vi "Calc_frequency.vi"(0 "ExitationTime In":dbl, 1 "X-length":dbl, 5 "CamTolerance":dbl=1.1, 9 "frequency in":dbl=5000.0, 11 "error in":errorcluster, 12 "X-Delta":dbl) -> (2 "Wavepoints":dbl, 3 "N":dbl=8192.0, 4 "TriggerLineCamWavepoints":dbl[](array[numeric]), 6 "divisor out":i32, 8 "Array":u8[](array[numeric]), 15 "error out":errorcluster)   [LabVIEW 2011]
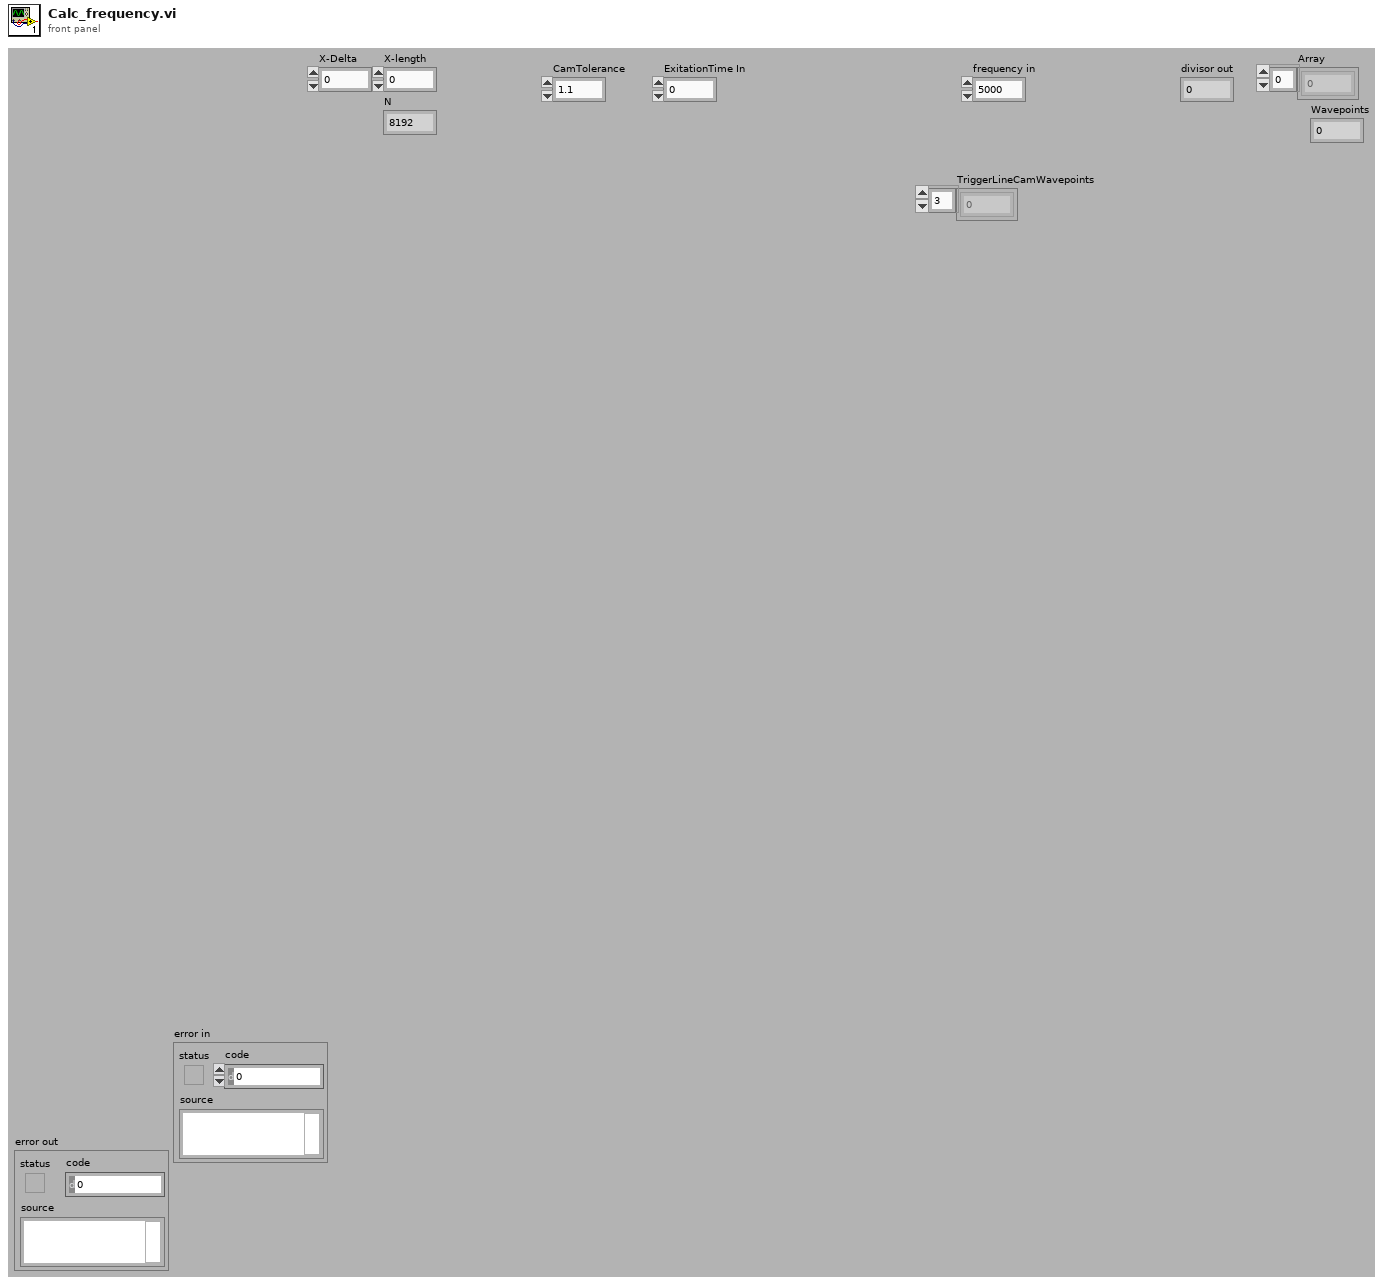
[diagram p1: front panel]
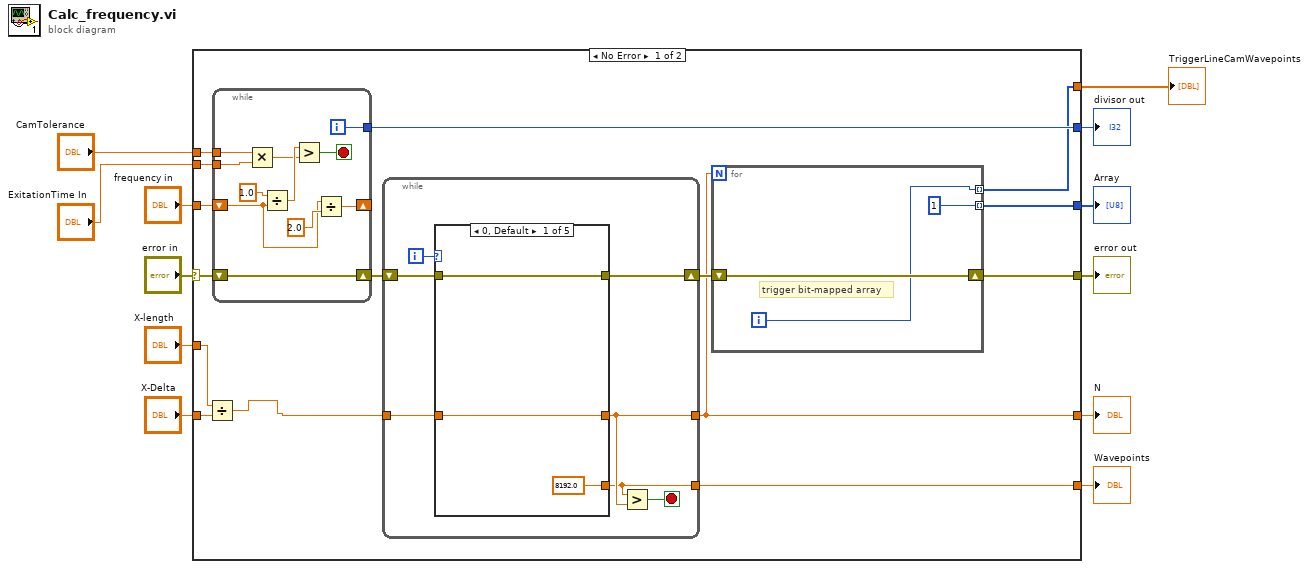
[diagram p0: block diagram]
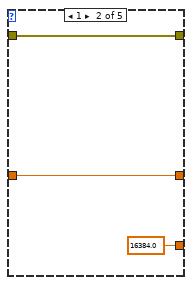
[diagram p2: hidden frame]
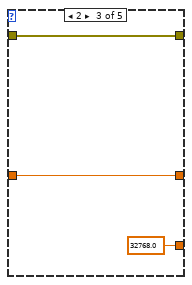
[diagram p3: hidden frame]
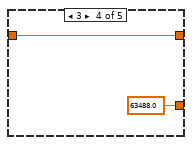
[diagram p4: hidden frame]
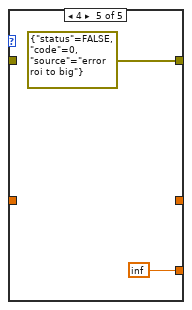
[diagram p5: hidden frame]
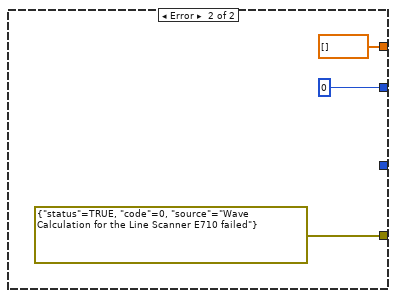
[diagram p6: hidden frame]
diagram:
  n1 = case shown="No Error" "error in" {
    selector: "error in" -> [w26 _]
    tunnel: "frequency in" -> [w22 _]
    tunnel: "CamTolerance" -> [w21 _]
    tunnel: "ExitationTime In" -> [w20 _]
    tunnel: [w27 errorcluster {"status"=TRUE, "code"=0, "source"="Wave Calculation for the Line Scanner E710 failed"} ("error IO")] -> w7
    tunnel: [w19 0] -> w10
    tunnel: [w14 dbl[] []] -> w8
    tunnel: [w25 _] -> w6
    tunnel: "X-Delta" -> [w23 _]
    tunnel: "X-length" -> [w24 _]
    tunnel: [w15 _] -> w1
    tunnel: [w16 _] -> w2
    frame No Error {
      n2 = Divide(x=w24, y=w23) -> (x/y=w13:dbl)
      n3 = while {
        shift-right: [w53] -> w17
        shift-left: w26 -> [w53]
        shift-right: [w50] -> _
        shift-left: w22 -> [w48]
        tunnel: w21 -> [w56]
        tunnel: w20 -> [w57]
        tunnel: [w51] -> w19
        i -> [w51]
        stop <- w52 stop-if-true
        n4 = Multiply(x=w56, y=w57) -> (x*y=w54:dbl)
        n5 = Divide(x=1.0, y=w48) -> (x/y=w55:dbl)
        n6 = Greater?(x=w55, y=w54) -> (0:w52:bool)
        n7 = Divide(x=w48, y=2.0) -> (x/y=w50:dbl)
      }
      n8 = while {
        tunnel: w13 -> [w30]
        shift-right: [w32] -> w18
        shift-left: w17 -> [w31]
        tunnel: [w29] -> w15
        tunnel: [w28] -> w16
        i -> [w34]
        stop <- w33 stop-if-true
        n9 = case shown="0, Default" w34 {
          tunnel: [8192.0 ("x") 16384.0 ("x") 32768.0 ("x") 63488.0 ("x") inf] -> w28
          tunnel: [w36 w39 w42 _ errorcluster {"status"=FALSE, "code"=0, "source"="error roi to big"} ("error IO")] -> w32
          tunnel: w31 -> [w36 w39 w42 _ _]
          tunnel: [w35 w38 w41 w44 _] -> w29
          tunnel: w30 -> [w35 w38 w41 w44 _]
          frame 0, Default {
          }
          frame 1 {
          }
          frame 2 {
          }
          frame 3 {
          }
          frame 4 {
          }
        }
        n10 = Greater?(x=w28, y=w29) -> (0:w33:bool)
      }
      n11 = for {
        N: w15 -> [_]
        shift-right: [w61] -> w27
        shift-left: w18 -> [w61]
        tunnel: [u8 1] -> w25 mode=indexing
        tunnel: [w59] -> w14 mode=indexing
        i -> [w59]
        # "trigger bit-mapped array"
      }
    }
    frame Error {
    }
  }
  "divisor out" <- w10
  "error out" <- w7
  "TriggerLineCamWavepoints" <- w8
  "Array" <- w6
  "N" <- w1
  "Wavepoints" <- w2
